vi "(SUBVI) - Turn Left Time.vi"(8 "NXT/EV3":T1, 10 "Time walking":dbl, 11 "Walk Speed":dbl) -> (0 "NXT/EV3 2":T1)   [LabVIEW 2016, in "testrobot.lvrbt"]
uses:
  testrobot.lvrbt
  <vilib>/NXT/Subs/LVHSConnector.ctl
  <vilib>/NXT/LegoClasses/BrickReference/BrickReference.lvclass
  <vilib>/NXT/Block Support/NXT_OutputPort.ctl
  <vilib>/NXT/NXTIO Xnodes/AddressXNode/NXTIOAddress.xnode
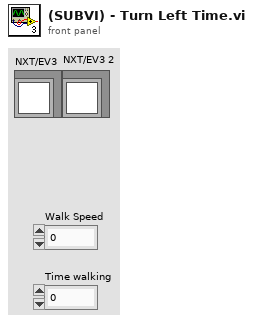
[diagram p1: front panel]
types:
  T1 = typedef "LVHSConnector.ctl" = refnum<class "BrickReference.lvclass">
  T2 = typedef "NXT_OutputPort.ctl" = u8
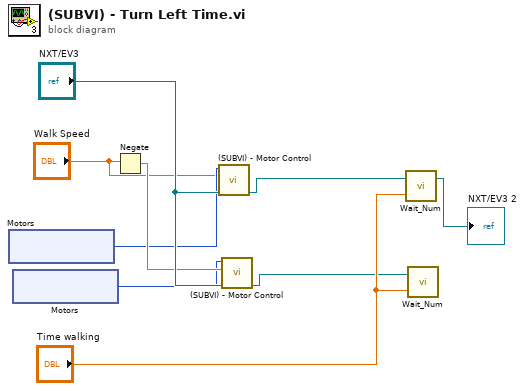
[diagram p0: block diagram]
diagram:
  n1 = xnode "Motors"() -> ("Motor"=w6:T2)
  n2 = xnode "Motors"() -> ("Motor"=w5:T2)
  n3 = Negate(x="Walk Speed") -> (-x=w7:dbl)
  n4 = call "(SUBVI) - Motor Control.vi"("NXT/EV3"="NXT/EV3", "Speed"="Walk Speed", "Motors"=w6) -> ("NXT/EV3 2"=w3:T1)  [unwired: 8 in]
  n5 = call "(SUBVI) - Motor Control.vi"("NXT/EV3"="NXT/EV3", "Speed"=w7, "Motors"=w5) -> ("NXT/EV3 2"=w2:T1)  [unwired: 8 in]
  n6 = call <vilib>:"Wait_Num.vi"("Time (1 sec)"="Time walking", "NXT/EV3"=w3) -> ("NXT/EV3"=→"NXT/EV3 2":T1)  [unwired: 2 in]
  n7 = call <vilib>:"Wait_Num.vi"("Time (1 sec)"="Time walking", "NXT/EV3"=w2) -> ()  [unwired: 2 in, 1 out]
